vi "Find Center Setup.vi"(0 "Carrier Tray":T1, 1 "Tray Number":dbl format="%#_13g", 2 "Position":i32, 3 "Assembly Type":string) -> (7 "Assembly Tray Out":T1)   [LabVIEW 2021, in "Assembly Tray.lvclass"]
uses:
  Assembly Tray.lvclass
  Find Tray.ctl
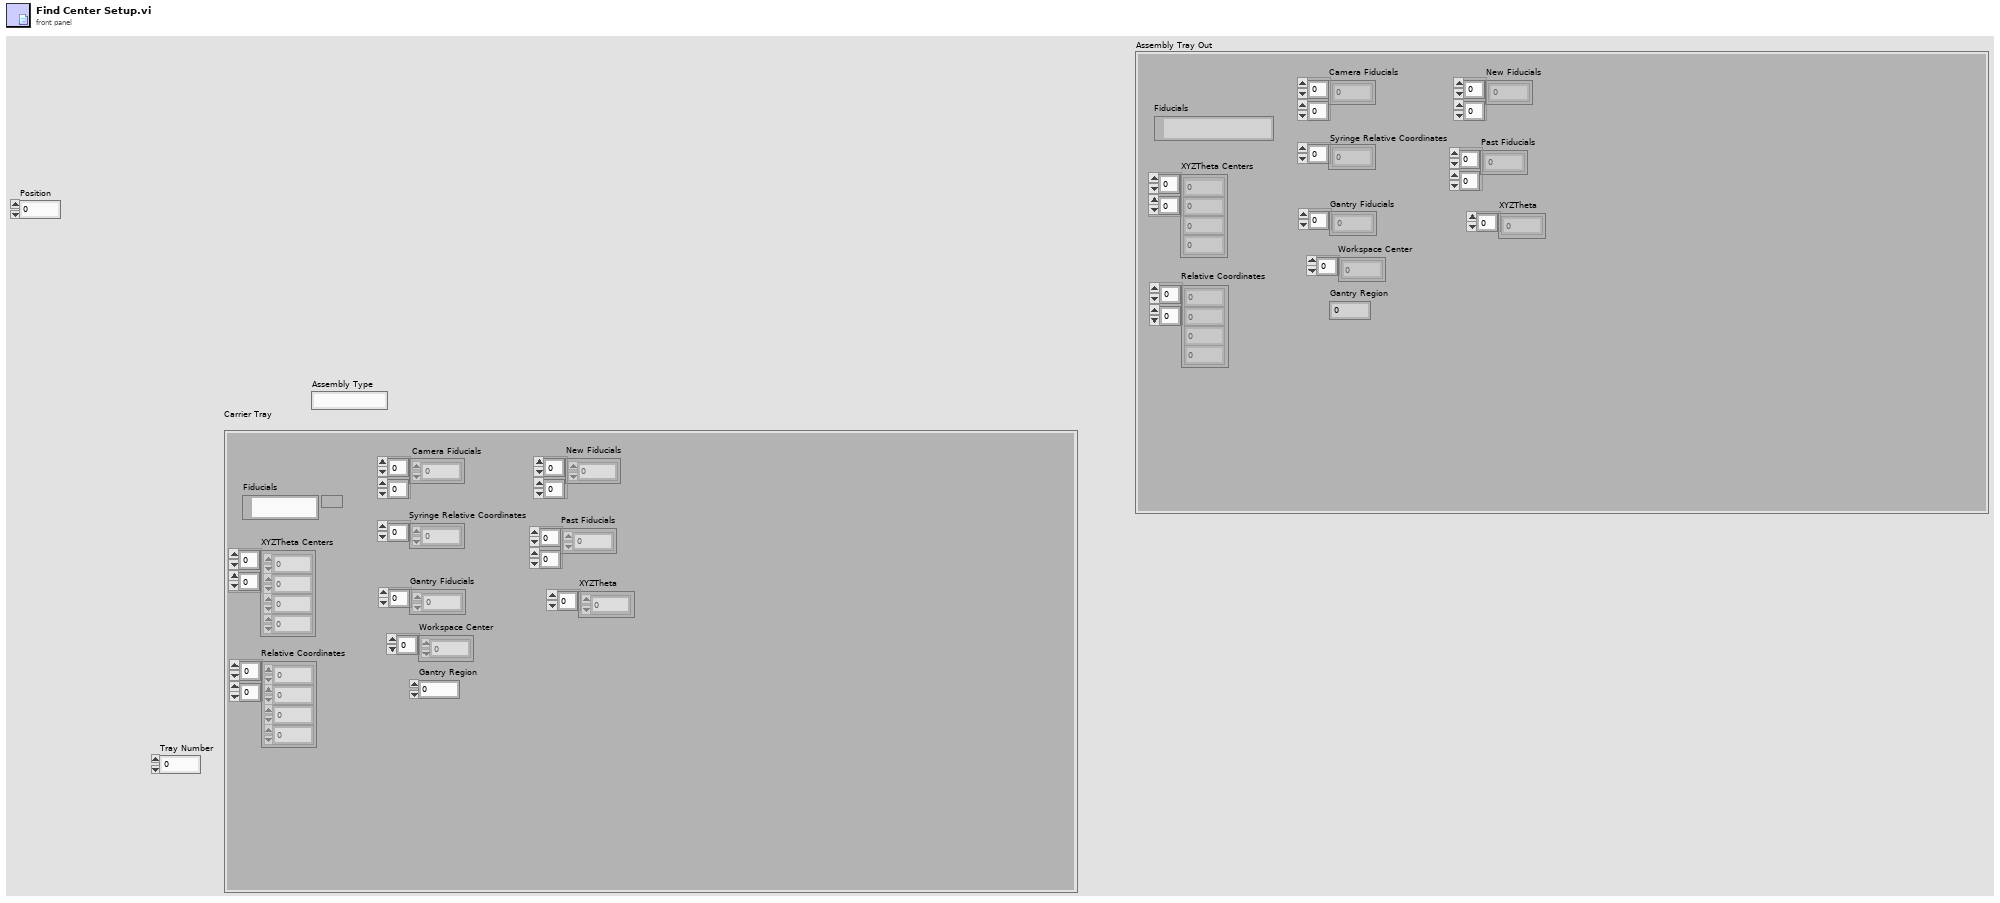
[diagram p1: front panel]
types:
  T1 = typedef "Assembly Tray.lvclass/Find Tray.ctl" = cluster{"Gantry Fiducials":dbl[], "Relative Coordinates":dbl[][], "Camera Fiducials":dbl[][], "XYZTheta Centers":dbl[][], "Workspace Center":dbl[], "Syringe Relative Coordinates":dbl[], "Gantry Region":dbl, "Fiducials":path, "New Fiducials":dbl[][], "Past Fiducials":dbl[][], "XYZTheta":dbl[]}
  T2 = typedef "File Paths.ctl" = cluster{"Glue Pattern Folder":path, "Carrier Tray Folder":path, "Pick Up Tool Fixture Folder":path, "Components Folder":path, "Bellows Tool Offset.txt":path, "Pick Up Tool Offset.txt":path, "Dispense Tip Offset.txt":path, "Log Files":path, "Gantry Assembly Map.txt":path, "Syringe and offset map.txt":path, "Controllers Folder":path}
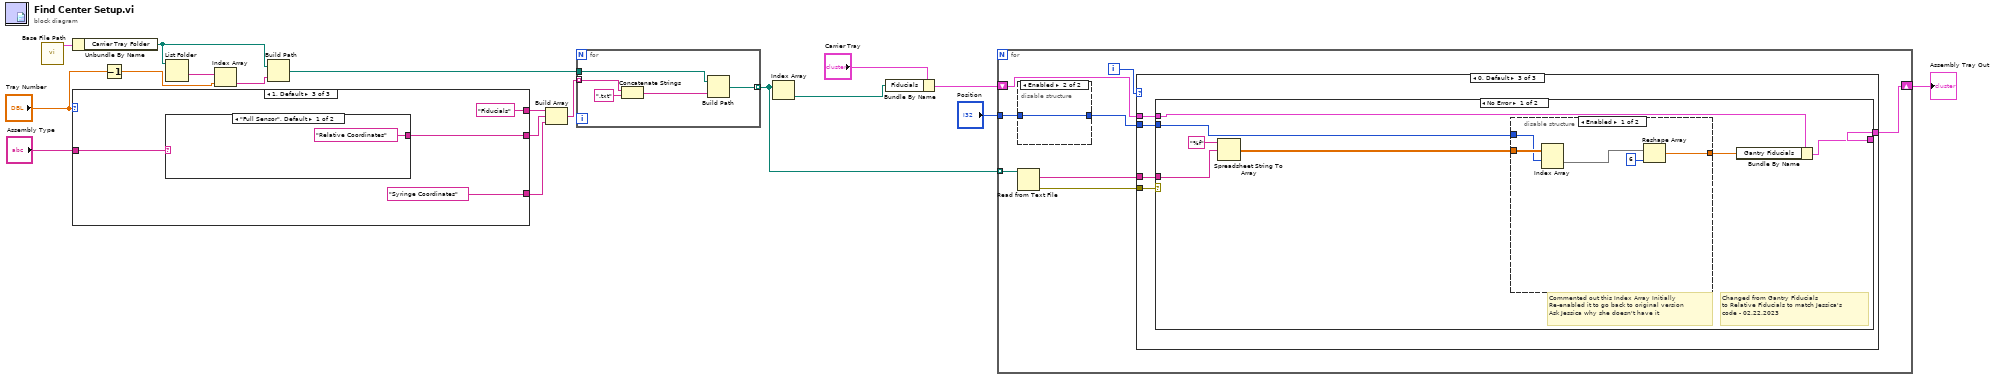
[diagram p0: block diagram]
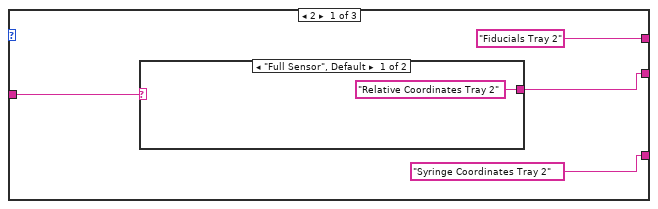
[diagram p2: hidden frame]
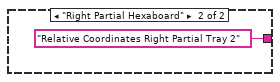
[diagram p3: hidden frame]
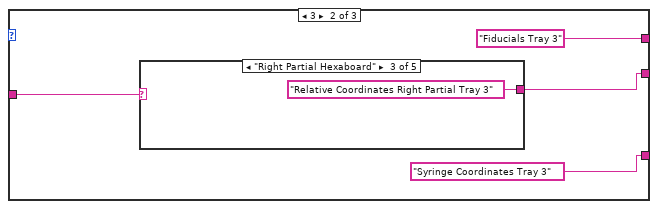
[diagram p4: hidden frame]
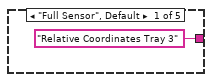
[diagram p5: hidden frame]
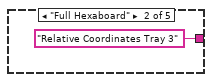
[diagram p6: hidden frame]
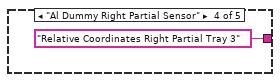
[diagram p7: hidden frame]
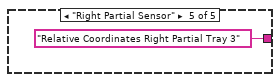
[diagram p8: hidden frame]
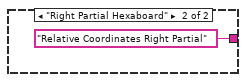
[diagram p9: hidden frame]
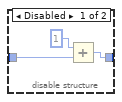
[diagram p10: hidden frame]
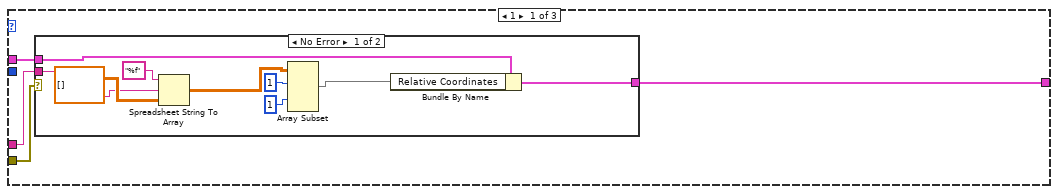
[diagram p11: hidden frame]
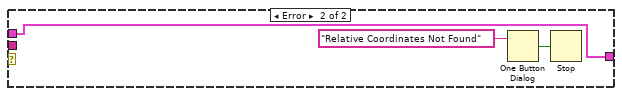
[diagram p12: hidden frame]
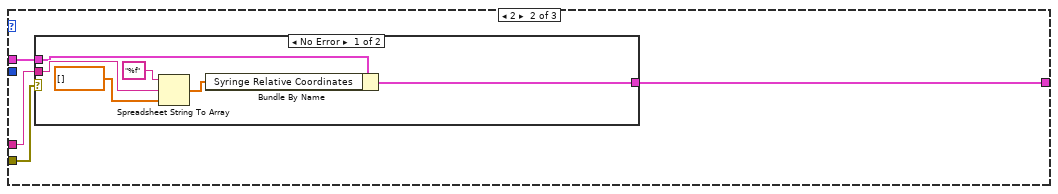
[diagram p13: hidden frame]
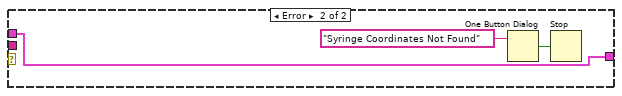
[diagram p14: hidden frame]
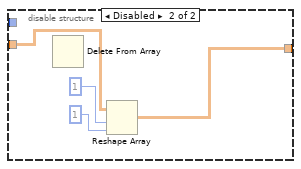
[diagram p15: hidden frame]
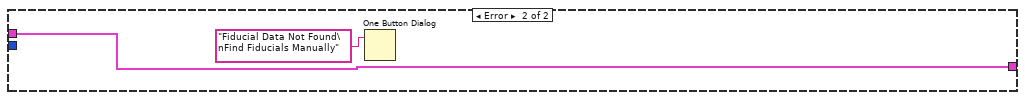
[diagram p16: hidden frame]
diagram:
  n1 = call "Base File Path.vi"() -> ("Paths Out"=w13:T2)  [unwired: 11 in]
  n2 = Unbundle By Name(w13) -> ("Carrier Tray Folder"=w6:path)
  n3 = case shown="1, Default" "Tray Number" {
    tunnel: [w21 w27 w37] -> w9
    tunnel: "Assembly Type" -> [w22 w28 w36]
    tunnel: ["Fiducials Tray 2" ("format string") "Fiducials Tray 3" ("format string") "Fiducials" ("format string")] -> w4
    tunnel: ["Syringe Coordinates Tray 2" ("element") "Syringe Coordinates Tray 3" ("element") "Syringe Coordinates" ("element")] -> w3
    frame 2 {
      n4 = case shown="\"Full Sensor\", Default" w22 {
        tunnel: ["Relative Coordinates Tray 2" ("format string") "Relative Coordinates Right Partial Tray 2" ("format string")] -> w21
        frame "Full Sensor", Default {
        }
        frame "Right Partial Hexaboard" {
        }
      }
    }
    frame 3 {
      n5 = case shown="\"Right Partial Hexaboard\"" w28 {
        tunnel: ["Relative Coordinates Tray 3" ("format string") "Relative Coordinates Tray 3" ("format string") "Relative Coordinates Right Partial Tray 3" ("format string") "Relative Coordinates Right Partial Tray 3" ("format string") "Relative Coordinates Right Partial Tray 3" ("format string")] -> w27
        frame "Full Sensor", Default {
        }
        frame "Full Hexaboard" {
        }
        frame "Right Partial Hexaboard" {
        }
        frame "Al Dummy Right Partial Sensor" {
        }
        frame "Right Partial Sensor" {
        }
      }
    }
    frame 1, Default {
      n6 = case shown="\"Full Sensor\", Default" w36 {
        tunnel: ["Relative Coordinates" ("format string") "Relative Coordinates Right Partial" ("format string")] -> w37
        frame "Full Sensor", Default {
        }
        frame "Right Partial Hexaboard" {
        }
      }
    }
  }
  n7 = Decrement(x="Tray Number") -> (x-1=w11:dbl)
  n8 = List Folder(path=w6) -> (folder names=w15:string[])  [unwired: 3 in, 3 out]
  n9 = Index Array "Index Array"(array=w15, index=w11) -> (element=w14:string)
  n10 = Build Path(base path=w6, name or relative path=w14) -> (appended path=w7:path)
  n11 = Build Array(w4, w9, w3) -> (w16:string[])
  n12 = for {
    tunnel: w16 -> [w43] mode=indexing
    tunnel: w7 -> [w44]
    tunnel: [w40] -> w8 mode=indexing
    n13 = Concatenate Strings "Concatenate Strings"(w43, ".txt" ("string")) -> (w41:string)
    n14 = Build Path(base path=w44, name or relative path=w41) -> (appended path=w40:path)
  }
  n15 = Index Array "Index Array"(array=w8) -> (element=w17:path)  [unwired: 1 in]
  n16 = Bundle By Name "Bundle By Name"(cluster="Carrier Tray", "Fiducials"=w17) -> (w18:T1)
  n17 = for {
    tunnel: w8 -> [w51] mode=indexing
    shift-right: [w47] -> w12
    shift-left: w18 -> [w48]
    tunnel: "Position" -> [w46]
    i -> [w49]
    n18 = disable-structure shown="Enabled" {
      disable-tunnel: w46 -> [w54 w56]
      disable-tunnel: [w53 w56] -> w45
      frame Disabled {
        n19 = Add(x=1, y=w54) -> (x+y=w53:i32)
      }
      frame Enabled {
      }
    }
    n20 = Read from Text File(file (use dialog)=w51) -> (text=w52:string, error out=w50:errorcluster)  [unwired: 3 in, 2 out]
    n21 = case shown="0, Default" w49 {
      tunnel: w52 -> [w59 w74 w90]
      tunnel: w50 -> [w60 w75 w89]
      tunnel: w48 -> [w58 w76 w88]
      tunnel: [w57 w73 w87] -> w47
      tunnel: w45 -> [_ _ w86]
      frame 1 {
        n22 = case shown="No Error" w60 {
          tunnel: w59 -> [w67 _]
          tunnel: [w65 w70] -> w57
          tunnel: w58 -> [w66 w70]
          frame No Error {
            n23 = Spreadsheet String To Array(format string="%f", spreadsheet string=w67, array type (2D Dbl)=dbl[][] []) -> (array=w64:dbl[][])  [unwired: 1 in]
            n24 = Array Subset(array=w64, index (row)=1 ("length"), index (col)=1 ("index (row)")) -> (w63:dbl[][])  [unwired: 2 in]
            n25 = Bundle By Name(cluster=w66, "Relative Coordinates"=w63) -> (w65:T1)
          }
          frame Error {
            n26 = One Button Dialog(message="Relative Coordinates Not Found") -> (true=w71:bool)  [unwired: 1 in]
            n27 = Stop(stop? (T)=w71) -> ()
          }
        }
      }
      frame 2 {
        n28 = case shown="No Error" w75 {
          tunnel: w74 -> [w80 _]
          tunnel: [w78 w83] -> w73
          tunnel: w76 -> [w79 w83]
          frame No Error {
            n29 = Spreadsheet String To Array(format string="%f", spreadsheet string=w80, array type (2D Dbl)=dbl[] []) -> (array=w77:dbl[])  [unwired: 1 in]
            n30 = Bundle By Name(cluster=w79, "Syringe Relative Coordinates"=w77) -> (w78:T1)
          }
          frame Error {
            n31 = One Button Dialog(message="Syringe Coordinates Not Found") -> (true=w84:bool)  [unwired: 1 in]
            n32 = Stop(stop? (T)=w84) -> ()
          }
        }
      }
      frame 0, Default {
        n33 = case shown="No Error" w89 {
          tunnel: w90 -> [w96 _]
          tunnel: w88 -> [w94 w107]
          tunnel: [w95 w107] -> w87
          tunnel: w86 -> [w91 _]
          frame No Error {
            # "Commented out this Index Array Initially\nRe-enabled it to go back to original version\nAsk Jessica why she doesn't have it"
            # "Changed from Gantry Fiducials\nto Relative Fiducials to match Jessica's \ncode - 02.22.2023"
            n34 = Spreadsheet String To Array(format string="%f", spreadsheet string=w96) -> (array=w92:dbl[][])  [unwired: 2 in]
            n35 = disable-structure shown="Enabled" {
              disable-tunnel: [w102 w103] -> w93
              disable-tunnel: w92 -> [w101 w106]
              disable-tunnel: w91 -> [w98 _]
              frame Enabled {
                n36 = Index Array "Index Array"(array=w101, index (row)=w98) -> (element=w100:dbl[])  [unwired: 1 in]
                n37 = Reshape Array "Reshape Array"(w100, 6 ("dimension size")) -> (w102:dbl[])
              }
              frame Disabled {
                n38 = Delete From Array "Delete From Array"() -> ()  [unwired: 3 in, 2 out]
                n39 = Reshape Array "Reshape Array"(w106, 1 ("dimension size"), 1 ("dimension size")) -> (w103:dbl[][])
              }
            }
            n40 = Bundle By Name "Bundle By Name"(cluster=w94, "Gantry Fiducials"=w93) -> (w95:T1)
          }
          frame Error {
            n41 = One Button Dialog(message="Fiducial Data Not Found\nFind Fiducials Manually") -> ()  [unwired: 1 in, 1 out]
          }
        }
      }
    }
  }
  "Assembly Tray Out" <- w12
